vi "Phasor Explorer Settings Window.vi"() -> ()   [LabVIEW 2019]
uses:
  Phasor Explorer Detector Parameters.ctl
  SEPXP Gate Parameter to Adjust.ctl
  Phasor Explorer Gate Parameters.ctl
  Gate Type.ctl
  Phasor Explorer Decay Parameters.ctl
  IRF Model.ctl
  Phasor Explorer Phasor Parameters.ctl
  Phasor Calculation Type.ctl
  Phasor Type.ctl
  Phasor Explorer Display Parameters.ctl
  Type of Series.ctl
  SEPXP Q [Element].ctl
  SEPXP Q [Event] List.ctl
panel:
  in  "Parameter Tabs":T1(tab)=enum."Gates"
  in  "Phasor Explorer Display Parameters":T2={"# Points"=1000, "Ramp Type"=enum."Logarithmic", "Type of Series"=enum."1-Exp Decays", "Min tau"=1.0000000000000002e-12, "Max tau"=1.0000000000000001e-07, "Include 0"=FALSE, "Include Infinity"=FALSE} {"Min tau" min=0.0; "Max tau" min=0.0; "# Points" min=1 step=1}
  out "f*":dbl[unit]=80000000.0 format="%#_5g"
  out "tau*":dbl[unit]=1.9894367886486918e-09 format="%#_5g"
  in  "Phasor Explorer Phasor Parameters":T4={"Harmonic frequency"=80000000.0, "Use f* = 1/D Frequency"=FALSE, "Calibrated Phasor"=FALSE, "Calibration Lifetime"=1e-09, "Phasor Calculation"=enum."Direct Sum", "SEPL Type"=enum."UC", "# Gates"=1.0, "Square Gate Width"=1e-09, "Show Ticks"=FALSE} {"Square Gate Width" min=0.0; "# Gates" min=0.0; "Calibration Lifetime" min=0.0; "Harmonic frequency" min=0.0}
  in  "Phasor Explorer Decay & IRF Parameters":T7={"Lifetime"=3.0000000000000004e-09, "IRF Offset"=0.0, "Laser Period"=1.2500000000000001e-08, "Normalized Decays"=FALSE, "IRF Model"=enum."Dirac", "IRF Parameter 1"=0.0} {"Lifetime" min=0.0; "Laser Period" min=0.0}
  in  "Edit User-defined Gate":bool
  in  "Gate Parameter to Adjust":T9 caption="Adjust"
  in  "Match Laser Period":bool=TRUE
  in  "Phasor Explorer Gate Parameters":T10={"First Gate Start"=0.0, "Use Gate Center"=FALSE, "Gate Width"=0.0, "Gate Step"=1.785714285714286e-09, "# Gates"=7.0, "Gate Type"=enum."Square", "Edge Width"=0.0, "Top Slope"=0.0, "Reversed Sawtooth?"=FALSE, "Analytical Computation"=FALSE, "Tolerance"=1.0, "Integration"=enum."Item 0", "# Steps"=1.0, "Type of User-defined Function"=enum."Gate"} {"# Steps" min=0.0; "Tolerance" min=0.0; "Top Slope" min=0.0; "Edge Width" min=0.0; "Gate Step" min=0.0; "# Gates" min=1.0 step=1.0; "Gate Width" min=0.0}
  in  "Phasor Explorer Detector Parameters":T12={"Frames/Image"=0, "Gates/Frame"=1, "Bits/Frame"=1, "Multiplicity"=0, "Incident Signal"=0.0} {"Frames/Image" min=1; "Multiplicity" min=0; "Bits/Frame" min=1; "Gates/Frame" min=1}
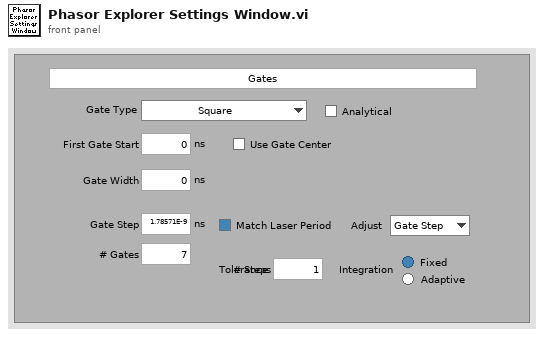
[diagram p1: front panel]
types:
  T1 = enum32{"Display", "Phasor", "Decay", "Gates", "Detector"}
  T2 = typedef "Phasor Explorer Display Parameters.ctl" = cluster{"# Points":i32, "Ramp Type":enum16{"Linear", "Logarithmic"}, "Type of Series":T3, "Min tau":dbl[unit], "Max tau":dbl[unit], "Include 0":bool, "Include Infinity":bool}
  T3 = typedef "Type of Series.ctl" = enum16{"1-Exp Decays", "Linear Combination of 1-Exp"}
  T4 = typedef "Phasor Explorer Phasor Parameters.ctl" = cluster{"Harmonic frequency":dbl[unit], "Use f* = 1/D Frequency":bool, "Calibrated Phasor":bool, "Calibration Lifetime":dbl[unit], "Phasor Calculation":T5, "SEPL Type":T6, "# Gates":dbl, "Square Gate Width":dbl[unit], "Show Ticks":bool}
  T5 = typedef "Phasor Calculation Type.ctl" = enum16{"Direct Sum", "Analytical Formula"}
  T6 = typedef "Phasor Type.ctl" = enum16{"UC", "L_N", "L_N[W]"}
  T7 = typedef "Phasor Explorer Decay Parameters.ctl" = cluster{"Lifetime":dbl[unit], "IRF Offset":dbl[unit], "Laser Period":dbl[unit], "Normalized Decays":bool, "IRF Model":T8, "IRF Parameter 1":dbl[unit]}
  T8 = typedef "IRF Model.ctl" = enum16{"Dirac", "Exponential"}
  T9 = typedef "SEPXP Gate Parameter to Adjust.ctl" = enum16{"Gate Step", "# Gates"}
  T10 = typedef "Phasor Explorer Gate Parameters.ctl" = cluster{"First Gate Start":dbl[unit], "Use Gate Center":bool, "Gate Width":dbl[unit], "Gate Step":dbl[unit], "# Gates":dbl, "Gate Type":T11, "Edge Width":dbl[unit], "Top Slope":dbl[unit], "Reversed Sawtooth?":bool, "Analytical Computation":bool, "Tolerance":dbl, "Integration":enum32{"Item 0", "Item 1"}, "# Steps":dbl, "Type of User-defined Function":enum32{"Gate", "IRF"}}
  T11 = typedef "Gate Type.ctl" = enum16{"Square", "Finite Edge Square", "Finite Edge, Tilted Top Square", "Triangle", "Sawtooth", "User-defined"}
  T12 = typedef "Phasor Explorer Detector Parameters.ctl" = cluster{"Frames/Image":i32, "Gates/Frame":i32, "Bits/Frame":i32, "Multiplicity":i32, "Incident Signal":dbl}
  T13 = typedef "SEPXP Q [Element].ctl" = cluster{"SEPXP Q Event":T14, "Data":variant}
  T14 = typedef "SEPXP Q [Event] List.ctl" = enum16{"Idle", "Initialization", "Show-Hide UC Ticks", "Edit User-defined Gate", "Update Phasor Graph", "Update Sum of Gates Graph", "Update Parameters", "Compute Decay &/or Gates", "Find Pseudo UC Intersections", "Compute alpha(beta) Plot", "Compute Pseudo-Phase Lifetime Plot", "Export Parameters to Clipboard", "Update Phase & Modulus Lifetime", "XY Graph Special Event", "Update Graph Plots Info", "Fit to Circle", "Quit"}
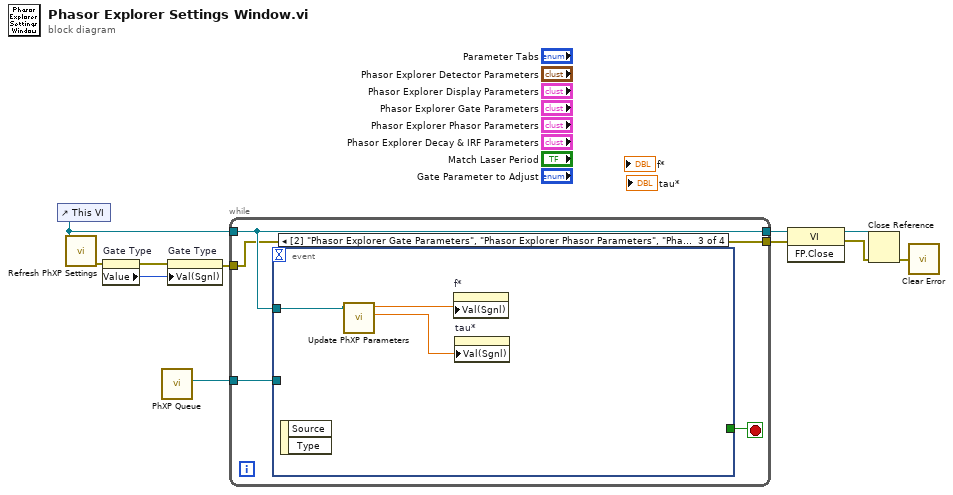
[diagram p0: block diagram]
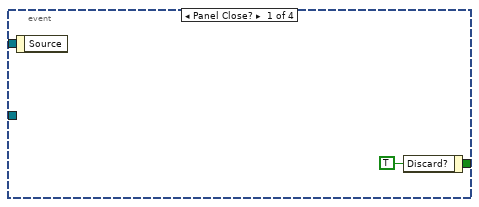
[diagram p2: hidden frame]
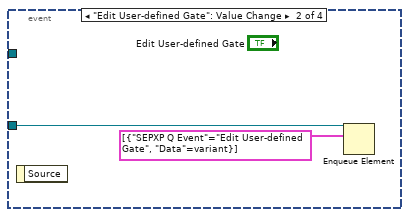
[diagram p3: hidden frame]
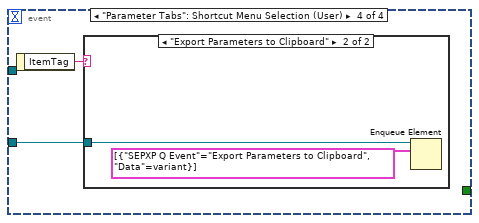
[diagram p4: hidden frame]
diagram:
  n1 = control-ref of="This VI"() -> (w3:refnum<vi>)
  n2 = call "Refresh PhXP Settings.vi"("VI in"=w3) -> ("error out"=w1:errorcluster)  [unwired: 10 in]
  n3 = property on="Gate Type" class="Enum (strict)"(error in=w1) -> (error out=w4:errorcluster, "Value"=w8:T11)  [unwired: 1 in, 1 out]
  n4 = call "PhXP Queue.vi"() -> ("PhXP Queue"=w9:refnum<queue>)  [unwired: 11 in]
  n5 = property on="Gate Type" class="Enum (strict)"(error in=w4, "Val(Sgnl)"=w8) -> (error out=w2:errorcluster)  [unwired: 1 in, 1 out]
  n6 = while {
    tunnel: [w14] -> w11
    tunnel: w2 -> [w12]
    tunnel: w9 -> [w13]
    tunnel: w3 -> [w14]
    tunnel: [w12] -> w5
    stop <- w15 stop-if-true
    n7 = event shown="[2] \"Phasor Explorer Gate Parameters\", \"Phasor Explorer Phasor Parameters\", \"Phasor Explorer Decay & IRF Parameters\", \"Phasor Explorer Display Parameters\", \"Match Laser Period\": Value Change" {
      selector: _ -> [_ _ _ _]
      dyn-events: _ -> [_ _ _ _]
      timeout: _ -> [_ _ _ _]
      tunnel: [w16 _ _ _] -> w15
      tunnel: w14 -> [_ _ w19 _]
      tunnel: w13 -> [_ w18 _ w22]
      event Panel Close? {
        w16 = TRUE ("Discard?")
        n8 = event-data() -> ()  [unwired: 1 in, 1 out]
        n9 = event-data("Discard?"=w16) -> ()  [unwired: 1 in, 1 out]
      }
      event "Edit User-defined Gate": Value Change {
        n10 = event-data() -> ()  [unwired: 1 in, 1 out]
        n11 = Enqueue Element(queue=w18, element=T13[] [{"SEPXP Q Event"=enum."Edit User-defined Gate", "Data"=variant}]) -> ()  [unwired: 2 in, 3 out]
      }
      event "Match Laser Period": Value Change {
        n12 = event-data() -> ()  [unwired: 1 in, 2 out]
        n13 = call "Update PhXP Parameters.vi"("VI in"=w19) -> ("tau*"=w20:dbl[unit], "f0"=w21:dbl[unit])  [unwired: 8 in, 1 out]
        n14 = property on="f*" class="DigNum (strict)"("Val(Sgnl)"=w21) -> ()  [unwired: 2 in, 2 out]
        n15 = property on="tau*" class="DigNum (strict)"("Val(Sgnl)"=w20) -> ()  [unwired: 2 in, 2 out]
      }
      event "Parameter Tabs": Shortcut Menu Selection (User) {
        n16 = event-data() -> ("ItemTag"=w23:string)  [unwired: 1 in]
        n17 = case shown="\"Export Parameters to Clipboard\"" w23 {
          tunnel: w22 -> [_ w25]
          frame "", Default {
          }
          frame "Export Parameters to Clipboard" {
            n18 = Enqueue Element(queue=w25, element=T13[] [{"SEPXP Q Event"=enum."Export Parameters to Clipboard", "Data"=variant}]) -> ()  [unwired: 2 in, 3 out]
          }
        }
      }
    }
  }
  n19 = invoke class="VI" method="FP.Close"(reference=w11, error in=w5) -> (reference out=w10:refnum<vi>, error out=w7:errorcluster)  [unwired: 1 in, 1 out]
  n20 = Close Reference(reference=w10, error in (no error)=w7) -> (error out=w6:errorcluster)
  n21 = call "Clear Error.vi"("Error In"=w6) -> ()  [unwired: 8 in, 1 out]
